vi "Variable@GetPointElement__Parameter.vi"(1 "ParamterIn":string) -> (0 "ParamterOut":string)   [LabVIEW 2019]
panel:
  in  "Axis":string(combo)
  in  "Point":string(combo)
  in  "Section":string(combo)
  in  "Variable":string(combo)
  in  "Confirm":bool
  # "Variable@GetPointElement $Variable=AXIS($Point)(,Section)\nAXIS is X,Y,Z,U,V,W,H"
  # "Variable=X(Point)(,Section)\nVariable=Y(Point)(,Section)\nVariable=Z(Point)(,Section)\nVariable=U(Point)(,Section)\nVariable=V(Point)(,Section)\nVariable=W(Point)(,Section)\nVariable=H(Point)(,Section)"
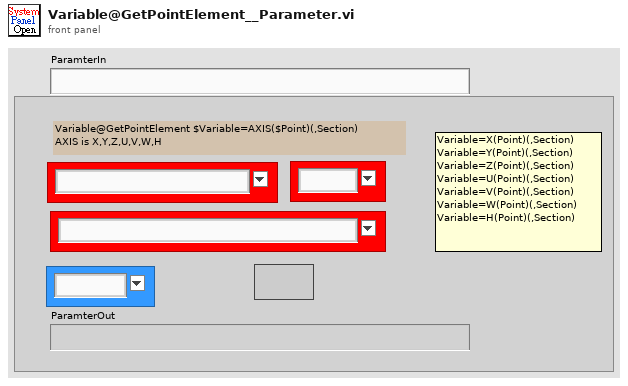
[diagram p1: front panel]
types:
  T1 = enum16{"Get", "UpdatePointS", "Init", "UpdateIndex", "GetCurrent&Index+1", "GetWithIndex", "ChkLast", "GetCurrent"}
  T2 = enum16{"Get", "Init", "Set", "Delete", "GetElement", "Inc", "Dec"}
  T3 = enum16{"Get", "Init", "Set", "Delete", "GetElement", "Inc", "Dec", "ReName"}
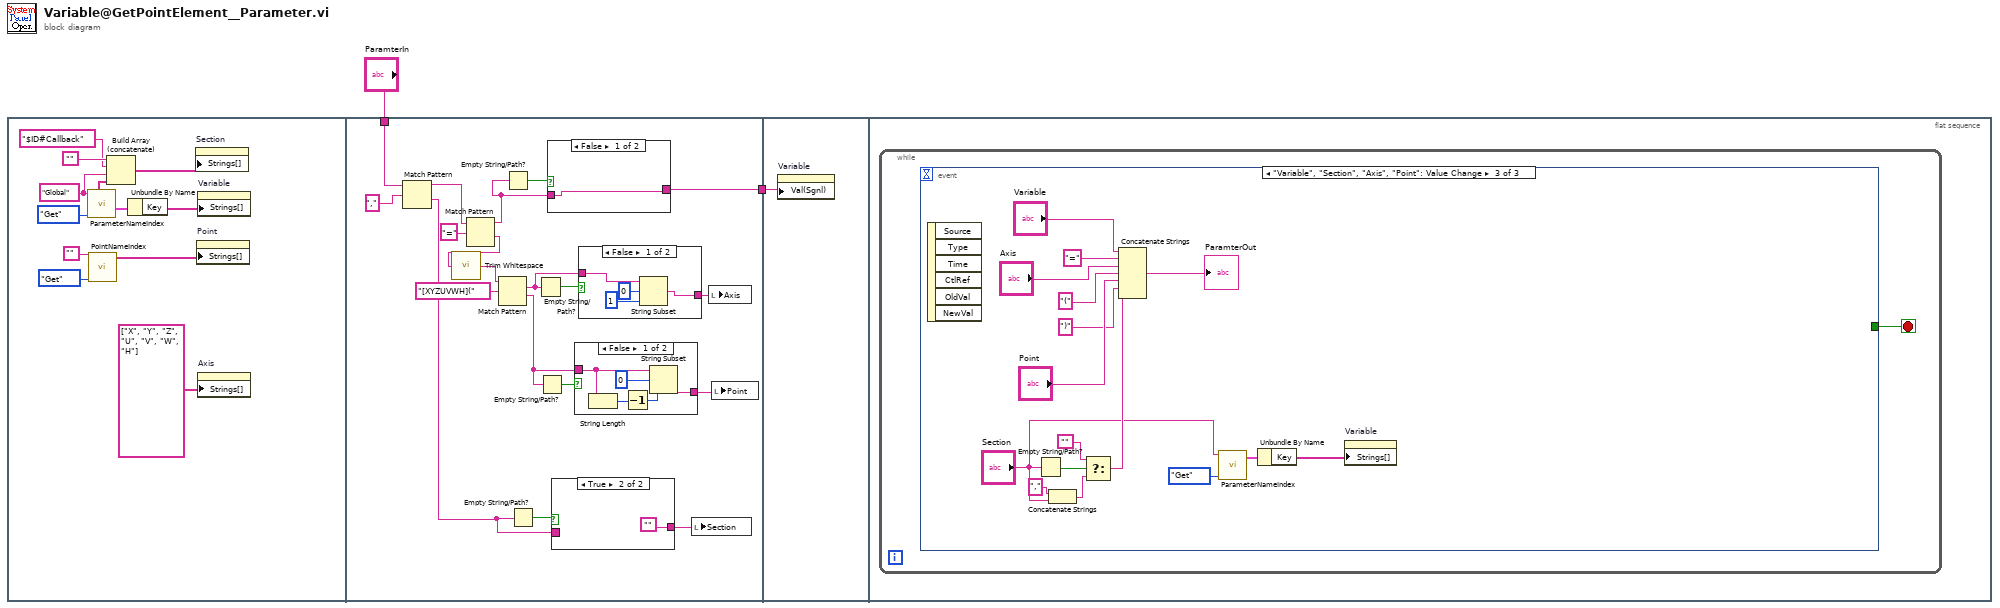
[diagram p0: block diagram]
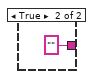
[diagram p2: hidden frame]
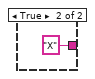
[diagram p3: hidden frame]
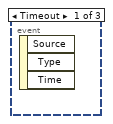
[diagram p6: hidden frame]
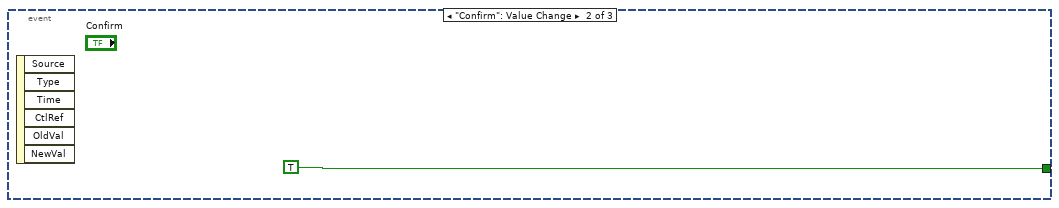
[diagram p7: hidden frame]
diagram:
  n1 = flat-sequence {
    tunnel: "ParamterIn" -> [w32]
    tunnel: [w28] -> w1
    tunnel: w1 -> [w49]
    frame #0 {
      w5 = "Global" ("VariableSection")
      n2 = call "ParameterNameIndex.vi"("OP"=T2."Get", "VariableSection"=w5) -> ("GlobalKeyValue"=w13:cluster{"Key":string[], "Value":string[]}, "SectionList"=w6:string[])  [unwired: 3 in, 5 out]
      n3 = call "PointNameIndex.vi"("OP"=T1."Get", "PointName"="") -> ("PointNameList"=w9:string[])  [unwired: 4 in, 5 out]
      n4 = Build Array (concatenate)("", "$ID#Callback" ("VariableSection"), w5, w6) -> (w4:string[])
      n5 = Unbundle By Name(w13) -> ("Key"=w12:string[])
      n6 = property on="Section" class="CmbBox"("Strings[]"=w4) -> ()  [unwired: 2 in, 2 out]
      n7 = property on="Point" class="CmbBox"("Strings[]"=w9) -> ()  [unwired: 2 in, 2 out]
      n8 = property on="Variable" class="CmbBox"("Strings[]"=w12) -> ()  [unwired: 2 in, 2 out]
      n9 = property on="Axis" class="CmbBox"("Strings[]"=string[] ["X", "Y", "Z", "U", "V", "W", "H"] ("Strings []")) -> ()  [unwired: 2 in, 2 out]
    }
    frame #1 {
      n10 = Match Pattern(string=w32, regular expression=",") -> (before substring=w26:string, after substring=w29:string)  [unwired: 1 in, 2 out]
      n11 = Match Pattern(string=w26, regular expression="=") -> (before substring=w23:string, after substring=w20:string)  [unwired: 1 in, 2 out]
      n12 = call <vilib>:"Trim Whitespace.vi"("string"=w20) -> ("trimmed string"=w19:string)  [unwired: 1 in]
      n13 = Match Pattern(string=w19, regular expression="[XYZUVWH](") -> (match substring=w18:string, after substring=w16:string)  [unwired: 1 in, 2 out]
      n14 = Empty String/Path?(string/path=w23) -> (empty?=w33:bool)
      n15 = Empty String/Path?(string/path=w29) -> (empty?=w30:bool)
      n16 = Empty String/Path?(string/path=w18) -> (empty?=w22:bool)
      n17 = Empty String/Path?(string/path=w16) -> (empty?=w17:bool)
      n18 = case shown="False" w33 {
        tunnel: w23 -> [w47 w48]
        tunnel: [w47 w48] -> w28
        frame False {
        }
        frame True {
        }
      }
      n19 = case shown="True" w30 {
        tunnel: w29 -> [w45 _]
        tunnel: [w45 ""] -> w27
        frame False {
        }
        frame True {
        }
      }
      n20 = case shown="False" w17 {
        tunnel: [w38 "" ("ParamterIn")] -> w15
        tunnel: w16 -> [w36 _]
        frame False {
          n21 = String Length(string=w36) -> (length=w35:i32)
          n22 = Decrement(x=w35) -> (x-1=w34:i32)
          n23 = String Subset(string=w36, offset (0)=0, length (rest)=w34) -> (substring=w38:string)
        }
        frame True {
        }
      }
      n24 = case shown="False" w22 {
        tunnel: [w41 "X" ("ParamterIn")] -> w21
        tunnel: w18 -> [w40 _]
        frame False {
          n25 = String Subset(string=w40, offset (0)=0, length (rest)=1 ("length (rest)")) -> (substring=w41:string)
        }
        frame True {
        }
      }
      n26 = local write "Section"(w27) -> ()
      n27 = local write "Axis"(w21) -> ()
      n28 = local write "Point"(w15) -> ()
    }
    frame #2 {
      n29 = property on="Variable" class="CmbBox"("Val(Sgnl)"=w49) -> ()  [unwired: 2 in, 2 out]
    }
    frame #3 {
      n30 = while {
        stop <- w50 stop-if-true
        n31 = event shown="[2] \"Variable\", \"Section\", \"Axis\", \"Point\": Value Change" {
          selector: _ -> [_ _ _]
          dyn-events: _ -> [_ _ _]
          timeout: _ -> [_ _ _]
          tunnel: [_ TRUE _] -> w50
          event Timeout {
            n32 = event-data() -> ()  [unwired: 1 in, 3 out]
          }
          event "Confirm": Value Change {
            n33 = event-data() -> ()  [unwired: 1 in, 6 out]
          }
          event "Variable", "Section", "Axis", "Point": Value Change {
            n34 = event-data() -> ()  [unwired: 1 in, 6 out]
            n35 = Empty String/Path?(string/path="Section") -> (empty?=w65:bool)
            n36 = Concatenate Strings("," ("string"), "Section") -> (w63:string)
            n37 = Select(t="", s=w65, f=w63) -> (s? t:f=w57:string)
            n38 = Concatenate Strings("Variable", "=" ("string"), "Axis", "(" ("string"), "Point", ")" ("string"), w57) -> (→"ParamterOut":string)
            n39 = call "ParameterNameIndex.vi"("OP"=T3."Get", "VariableSection"="Section") -> ("SectionKeyValue"=w53:cluster{"Key":string[], "Value":string[]})  [unwired: 3 in, 6 out]
            n40 = Unbundle By Name(w53) -> ("Key"=w55:string[])
            n41 = property on="Variable" class="CmbBox"("Strings[]"=w55) -> ()  [unwired: 2 in, 2 out]
          }
        }
      }
    }
  }
